vi "G4SubTemplate_Singleton_6x8x6_CleanUp.vi"(5 "Error In":errorcluster) -> (19 "Error Out":errorcluster)   [LabVIEW 2020, in "G4SubTemplate_Singleton_6x8x6.lvclass"]
uses:
  <resource>/Framework/Providers/Open_GDS/ClassProviders/Provider_EndevoGOOP400/Templates/G4SubTemplate_Singleton_6x8x6/G4SubTemplate_Singleton_6x8x6.lvclass
  <resource>/Framework/Providers/Open_GDS/ClassProviders/Provider_EndevoGOOP400/Templates/G4BaseTemplate_Singleton_6x8x6/G4BaseTemplate_Singleton_6x8x6.lvclass
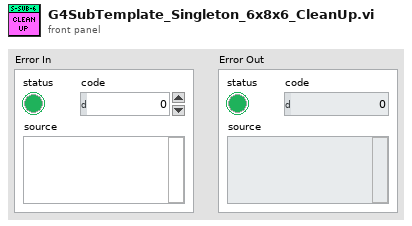
[diagram p1: front panel]
types:
  T1 = typedef "G4SubTemplate_Singleton_6x8x6.lvclass/ObjectAttributes.ctl" = cluster{"Attribute1":dbl}
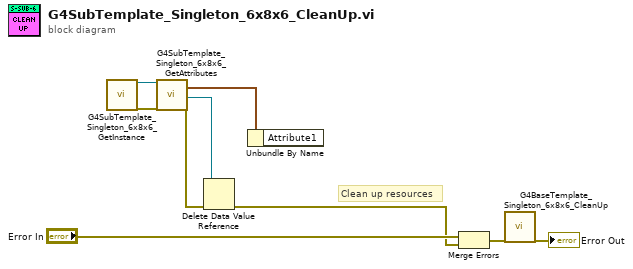
[diagram p0: block diagram]
diagram:
  # "Clean up resources"
  n1 = call <resource>:"G4SubTemplate_Singleton_6x8x6_GetInstance.vi"() -> ("reference out"=w7:refnum<class "G4SubTemplate_Singleton_6x8x6.lvclass">, "error out"=w8:errorcluster)  [unwired: 15 in, 3 out]
  n2 = call <resource>:"G4SubTemplate_Singleton_6x8x6_GetAttributes.vi"("reference in"=w7, "error in (no error)"=w8) -> ("Data"=w9:T1, "DataRef"=w3:refnum<data-value>, "error out"=w4:errorcluster)  [unwired: 14 in, 1 out]
  n3 = Delete Data Value Reference(data value reference=w3, error in=w4) -> (error out=w1:errorcluster)  [unwired: 1 out]
  n4 = Unbundle By Name(w9) -> ()  [unwired: 1 out]
  n5 = Merge Errors("Error In", w1) -> (w6:errorcluster)
  n6 = call <resource>:"G4BaseTemplate_Singleton_6x8x6_CleanUp.vi"("Error In"=w6) -> ("Error Out"=→"Error Out":errorcluster)  [unwired: 18 in]
